vi "Offset Change Message DAO.vi"(8 "error in (no error)":errorcluster, 9 "Offset In":T2, 11 "DAO Actions":T1=enum."Get") -> (0 "error out":errorcluster, 1 "Offset Out":T2, 4 "Notifier Name":string="Offset Status Change")   [LabVIEW 2009]
uses:
  Offset Message Type.ctl
  Data Access Objects/Metadata/DAO Actions.ctl
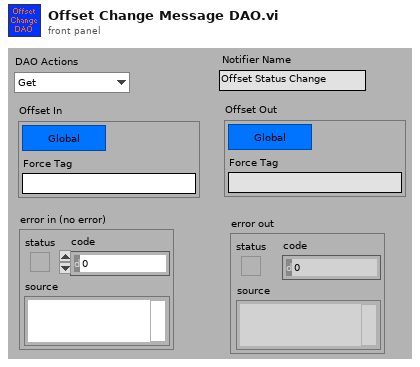
[diagram p1: front panel]
types:
  T1 = typedef "DAO Actions.ctl" = enum16{"Init", "Get", "Set"}
  T2 = typedef "Offset Message Type.ctl" = cluster{"Cartesian Type":bool, "Force Tag":string}
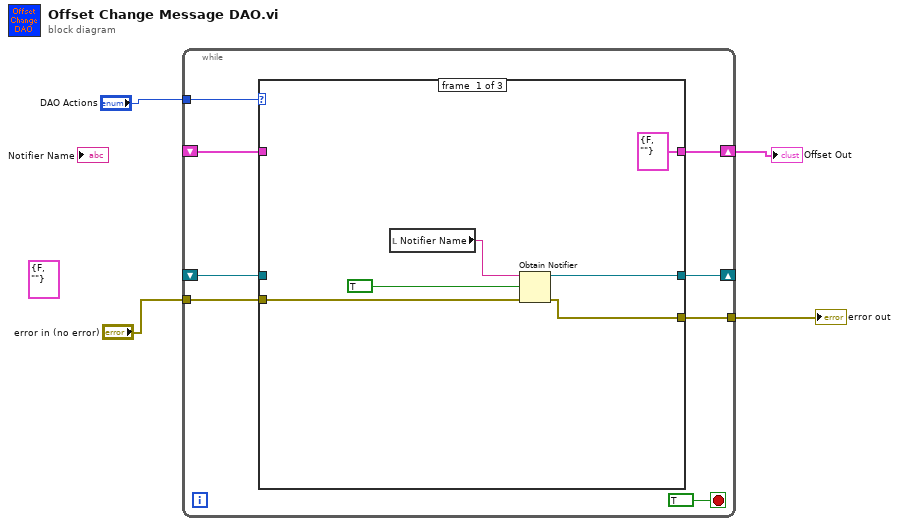
[diagram p0: block diagram]
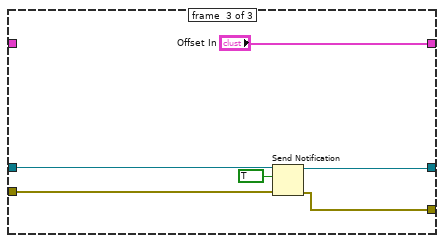
[diagram p3: hidden frame]
diagram:
  (unwired) T2 {"Cartesian Type"=FALSE, "Force Tag"=""} ("Offset In")
  n1 = while {
    tunnel: "DAO Actions" -> [w12]
    tunnel: "error in (no error)" -> [w11]
    tunnel: [w10] -> w2
    shift-right: [w9] -> _
    shift-left: _ -> [w7]
    shift-right: [w8] -> w1
    shift-left: _ -> [w6]
    stop <- TRUE stop-if-true
    n2 = case shown="\"Init\"" w12 {
      tunnel: w11 -> [w17 w19 w25]
      tunnel: [w16 w19 w24] -> w10
      tunnel: [w14 w20 w23] -> w9
      tunnel: [T2 {"Cartesian Type"=FALSE, "Force Tag"=""} ("Offset In") w21 "Offset In"] -> w8
      tunnel: w7 -> [_ w20 w26]
      tunnel: w6 -> [_ w21 _]
      frame #0 {
        n3 = local read "Notifier Name"() -> (w18:string)
        n4 = Obtain Notifier(name (unnamed)=w18, notification data type=TRUE, error in (no error)=w17) -> (notifier out=w14:refnum<notifier>, error out=w16:errorcluster)  [unwired: 1 in, 1 out]
      }
      frame #1 {
      }
      frame #2 {
        n5 = Send Notification(notification=TRUE, notifier=w26, error in (no error)=w25) -> (notifier out=w23:refnum<notifier>, error out=w24:errorcluster)
      }
    }
  }
  "Offset Out" <- w1
  "error out" <- w2
